vi "ArcadeDriveTest.vi"() -> ()   [LabVIEW 2013]
uses:
  <vilib>/Rock Robotics/WPI/Joystick/WPI_JoystickDeviceEnum.ctl
  <vilib>/Rock Robotics/SystemInterfaces/DIO/FPGA_DIOPWMChannel.ctl
  <vilib>/Rock Robotics/WPI/RobotDrive/WPI_RobotDriveOpen4MotorWithTalon.vi
  ArcadeDriveLinear.vi
  <vilib>/Rock Robotics/WPI/RobotDrive/WPI_RobotDriveArcadeDrive_Standard(NoSaturation).vi
panel:
  in  "Deadzone":dbl=0.05 format="%#_13g"
  in  "UseWPILib?":bool
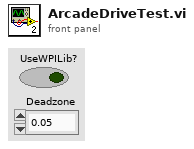
[diagram p1: front panel]
types:
  T1 = typedef "FPGA_DIOPWMChannel.ctl" = enum8{"PWM 1", "PWM 2", "PWM 3", "PWM 4", "PWM 5", "PWM 6", "PWM 7", "PWM 8", "PWM 9", "PWM 10", "Invalid"}
  T2 = typedef "WPI_JoystickDeviceEnum.ctl" = enum16{"USB 1", "USB 2", "USB 3", "USB 4", "Kinect 1", "Kinect 2"}
  T3 = typedef "WPI_RobotDriveDevRef.ctl" = cluster{"DevStatus":errorcluster, "Motors[]":T4[], "Square Inputs":bool, "Max Output":dbl, "Isochronous":bool}
  T4 = typedef "WPI_MotorControlDeviceRef.ctl" = cluster{"DeviceStatus":errorcluster, "Type":enum16{"PWM", "CAN"}, "PWM":cluster{"Digital Module":T5, "PWM Channel":T1, "DeadBand":T6}, "CAN":cluster{"Device Number":u8, "Control Mode":T7, "Semaphore":T8, "Max Vout":dbl}, "Invert":bool, "TransformRef":T9, "InvTransformRef":T9}
  T5 = typedef "FPGA_TypedefDigitalModule.ctl" = enum16{"Digital Module 1", "Digital Module 2"}
  T6 = typedef "WPI_PWMDeadband.ctl" = cluster{"Name":string, "maxPositivePwm":i32, "minPositivePwm":i32, "centerPwm":i32, "maxNegativePwm":i32, "minNegativePwm":i32, "angularRange":u16}
  T7 = typedef "WPI_CANJaguar_ControlMode.ctl" = enum8{"Percent VBus", "Current", "Speed", "Position", "Voltage"}
  T8 = typedef "Semaphore RefNum" = refnum<k1>
  T9 = typedef "WPI_PWMTransform_ConPane.ctl" = refnum<vi>
  T10 = typedef "WPI_JoystickDevRef.ctl" = cluster{"Device":T2}
  T11 = cluster{"axis 1 (x)":dbl, "axis 2 (y)":dbl, "axis 3 (throttle)":dbl, "axis 4":dbl, "axis 5":dbl, "axis 6":dbl}
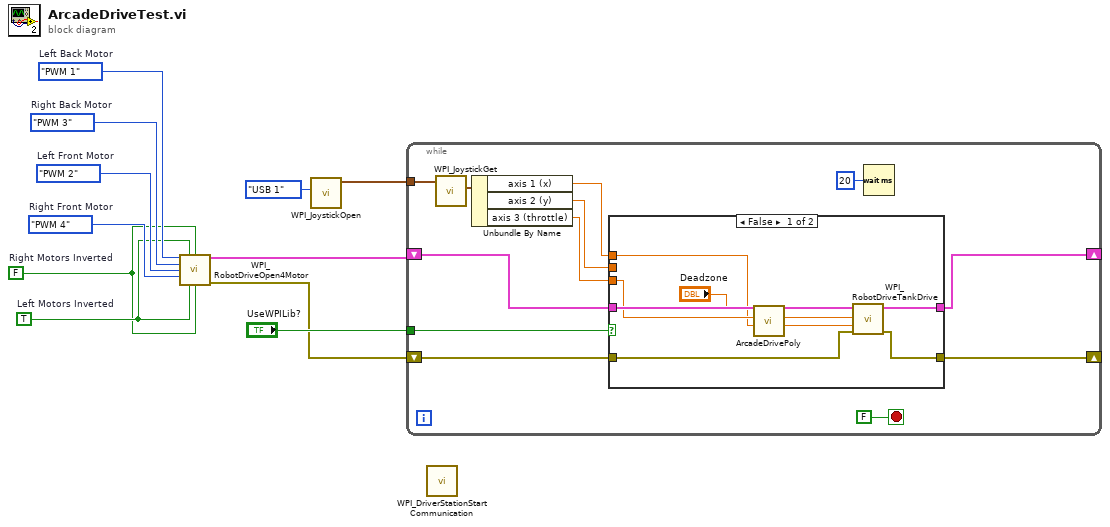
[diagram p0: block diagram]
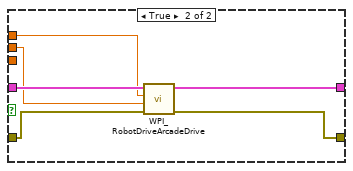
[diagram p2: hidden frame]
diagram:
  w5 = FPGA_DIOPWMChannel."PWM 4"  # Right Front Motor
  w6 = FPGA_DIOPWMChannel."PWM 2"  # Left Front Motor
  w7 = FPGA_DIOPWMChannel."PWM 3"  # Right Back Motor
  w8 = FPGA_DIOPWMChannel."PWM 1"  # Left Back Motor
  w3 = FALSE  # Right Motors Inverted
  w4 = TRUE  # Left Motors Inverted
  n1 = call-poly <vilib>:"WPI_RobotDriveOpen4Motor.vi"("Rear Left Motor"=w8, "Rear Left Motor Inverted"=w4, "Rear Right Motor Inverted"=w3, "Rear Right Motor"=w7, "Front Left Motor"=w6, "Front Right Motor"=w5, "Front Left Motor Inverted"=w4, "Front Right Motor Inverted"=w3) -> ("RobotDriveDevRef"=w2:T3, "error out"=w1:errorcluster)  [unwired: 6 in]
  n2 = call <vilib>:"WPI_JoystickOpen.vi"("JoystickDevice"=WPI_JoystickDeviceEnum."USB 1") -> ("JoystickDevRef"=w9:T10)  [unwired: 10 in]
  n3 = while {
    tunnel: "UseWPILib?" -> [w21]
    tunnel: w9 -> [w20]
    shift-right: [w12] -> _
    shift-left: w2 -> [w15]
    shift-right: [w13] -> _
    shift-left: w1 -> [w14]
    stop <- FALSE stop-if-true
    n4 = call <vilib>:"WPI_JoystickGet.vi"("JoystickDevRef"=w20) -> ("Axes"=w19:T11)  [unwired: 4 in, 2 out]
    n5 = Unbundle By Name(w19) -> ("axis 1 (x)"=w16:dbl, "axis 2 (y)"=w17:dbl, "axis 3 (throttle)"=w18:dbl)
    n6 = case shown="False" w21 {
      tunnel: w18 -> [w28 _]
      tunnel: w17 -> [_ w37]
      tunnel: w16 -> [w27 w36]
      tunnel: w15 -> [w32 w38]
      tunnel: w14 -> [w30 w35]
      tunnel: [w29 w34] -> w13
      tunnel: [w31 w33] -> w12
      frame False {
        n7 = call-poly "ArcadeDrivePoly.vi"("Direction"=w27, "Throttle"=w28, "Deadzone"="Deadzone") -> ("DriveRight"=w24:dbl, "DriveLeft"=w25:dbl)  [unwired: 7 in]
        n8 = call <vilib>:"WPI_RobotDriveTankDrive.vi"("error in (no error)"=w30, "Right axis value"=w24, "Left axis value"=w25, "RobotDriveDevRef"=w32) -> ("error out"=w29:errorcluster, "RobotDriveDevRef"=w31:T3)  [unwired: 5 in, 1 out]
      }
      frame True {
        n9 = call-poly <vilib>:"WPI_RobotDriveArcadeDrive.vi"("error in (no error)"=w35, "Y axis value"=w37, "X axis value"=w36, "RobotDriveDevRef"=w38) -> ("error out"=w34:errorcluster, "RobotDriveDevRef"=w33:T3)  [unwired: 5 in, 1 out]
      }
    }
    n10 = Wait (ms)(milliseconds to wait=u32 20) -> ()  [unwired: 1 out]
  }
  n11 = call <vilib>:"WPI_DriverStationStart Communication.vi"() -> ()  [unwired: 12 in]
